vi "LineCounterColor.vi"(7 "Port/MUX":T3 {"Port" items=["Port 1", "Port 2", "Port 3", "Port 4"]; "MUX Port" items=["No MUX", "MUX 1", "MUX 2", "MUX 3", "MUX 4"]}, 10 "Enum":T1, 11 "NXT In":T2) -> (2 "Numeric":i16, 3 "NXT Out":T2)   [LabVIEW 2012]
uses:
  <vilib>/NXT/Subs/LVHSConnector.ctl
  <vilib>/NXT/LegoClasses/BrickReference/BrickReference.lvclass
  <vilib>/NXT/HiTechnic/HiTechnic Controls/HiTechnic Port.ctl
  <vilib>/NXT/Block Support/NXT_InputPort.ctl
  LineCountColorCtl.ctl
  <vilib>/NXT/Block Support/NXT_TimerIndex.ctl
panel:
  out "Color":string="Black"
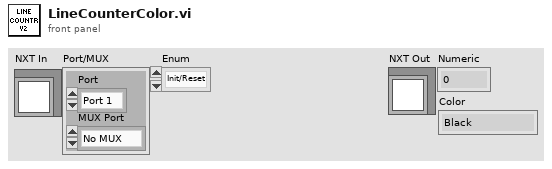
[diagram p1: front panel]
types:
  T1 = typedef "LineCountColorCtl.ctl" = enum16{"Init/Reset", "Check"}
  T2 = typedef "LVHSConnector.ctl" = refnum<class "BrickReference.lvclass">
  T3 = typedef "HiTechnic Port.ctl" = cluster{"Port":T4, "MUX Port":u8}
  T4 = typedef "NXT_InputPort.ctl" = u8
  T5 = typedef "NXT_TimerIndex.ctl" = u8
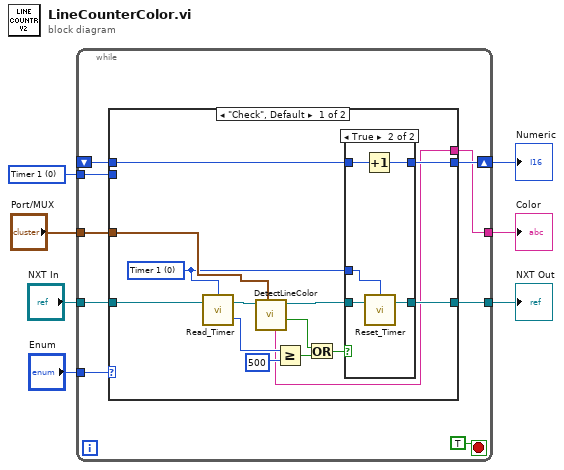
[diagram p0: block diagram]
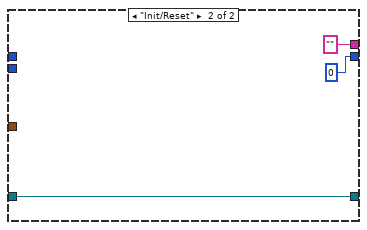
[diagram p3: hidden frame]
diagram:
  w1 = T5 0 items=["Timer 1", "Timer 2", "Timer 3"] ("Timer (Timer 1)")
  n1 = while {
    tunnel: "NXT In" -> [w16]
    tunnel: "Port/MUX" -> [w15]
    shift-right: [w13] -> w4
    shift-left: _ -> [w12]
    tunnel: [w11] -> w5
    tunnel: "Enum" -> [w10]
    tunnel: [w9] -> w2
    tunnel: w1 -> [w8]
    stop <- TRUE stop-if-true
    n2 = case shown="\"Check\", Default" w10 {
      tunnel: w16 -> [w29 w38]
      tunnel: w15 -> [w30 _]
      tunnel: [w18 i16 0] -> w13
      tunnel: w12 -> [w19 _]
      tunnel: [w20 w38] -> w11
      tunnel: [w17 "" ("Color")] -> w9
      tunnel: w8 -> [_ _]
      frame "Check", Default {
        w27 = T5 0 items=["Timer 1", "Timer 2", "Timer 3"] ("Timer (Timer 1)")
        n3 = call <vilib>:"Read_Timer.vi"("NXT"=w29, "Timer (Timer 1)"=w27) -> ("Value (msec)"=w26:u32, "NXT"=w28:T2)  [unwired: 1 in]
        n4 = call "DetectLineColor.vi"("Port/MUX"=w30, "NXT In"=w28) -> ("Detected Line?"=w23:bool, "NXT Out"=w21:T2, "Color"=w17:string)  [unwired: 7 in]
        n5 = Greater Or Equal?(x=w26, y=u32 500) -> (x >= y?=w24:bool)
        n6 = Or(x=w23, y=w24) -> (x .or. y?=w22:bool)
        n7 = case shown="True" w22 {
          tunnel: w27 -> [_ w37]
          tunnel: w21 -> [w31 w36]
          tunnel: [w31 w35] -> w20
          tunnel: w19 -> [w32 w34]
          tunnel: [w32 w33] -> w18
          frame False {
          }
          frame True {
            n8 = Increment(x=w34) -> (x+1=w33:i16)
            n9 = call <vilib>:"Reset_Timer.vi"("NXT"=w36, "Timer (Timer 1)"=w37) -> ("NXT"=w35:T2)  [unwired: 2 in]
          }
        }
      }
      frame "Init/Reset" {
      }
    }
  }
  "NXT Out" <- w5
  "Numeric" <- w4
  "Color" <- w2
